vi "read TDMS file -- wavefront -- V1.vi"(6 "Data type":waveform(dbl), 7 "tdms file in":refnum<k34>, 9 "Data File Type":T2(ring), 10 "Data window":T1={"Start"=0, "Length"=500000, "Channel numbers"=[0], "Channel name"="Vpick", "Group name"="p"}, 11 "Input file path":path) -> (1 "1st channel length":u64=433333, 2 "Data out":waveform(dbl), 3 "Actual input file path":path, 5 "tdms file out":refnum<k34>)   [LabVIEW 2021]
uses:
  tdo -- new/Data window.ctl
panel:
  # "OR"
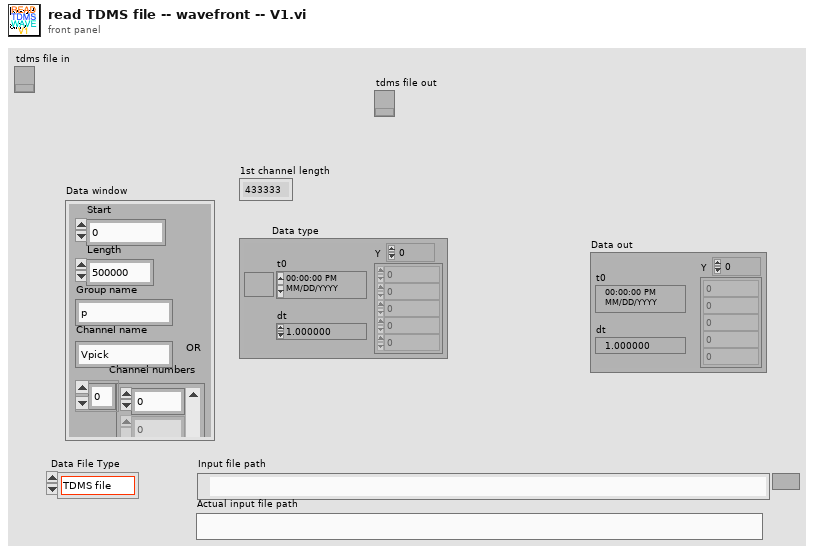
[diagram p1: front panel]
types:
  T1 = typedef "Data window.ctl" = cluster{"Start":i64, "Length":i64, "Channel numbers":i64[], "Channel name":string, "Group name":string}
  T2 = enum16{"TDMS file", "Tektronics ISF", "BinF file", "ASCII File", "BinH File", "BinW File", "BINARY File"}
  T3 = enum16{"open", "open or create", "create or replace", "create", "open (read-only)"}
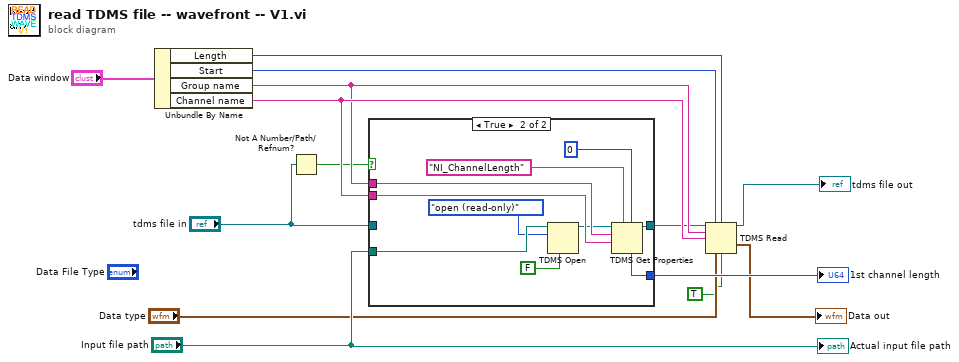
[diagram p0: block diagram]
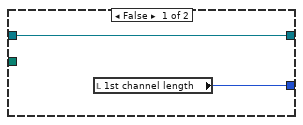
[diagram p2: hidden frame]
diagram:
  n1 = Unbundle By Name("Data window") -> ("Length"=w13:i64, "Start"=w4:i64, "Group name"=w10:string, "Channel name"=w12:string)
  n2 = Not A Number/Path/Refnum?(number/path/refnum="tdms file in") -> (NaN/Path/Refnum?=w2:bool)
  n3 = case shown="True" w2 {
    tunnel: [w16 w18] -> w3
    tunnel: "Input file path" -> [_ w26]
    tunnel: "tdms file in" -> [w16 _]
    tunnel: [w15 w22] -> w11
    tunnel: w12 -> [_ w21]
    tunnel: w10 -> [_ w20]
    frame False {
      n4 = local read "1st channel length"() -> (w15:u64)
    }
    frame True {
      n5 = TDMS Open(6:FALSE ("disable buffering (T)"), 10:T3."open (read-only)" ("operation (0:open)"), 11:w26) -> (3:w19:refnum<k34>)  [unwired: 4 in, 1 out]
      n6 = TDMS Get Properties(5:u64 0, 7:"NI_ChannelLength" ("property name"), 9:w21, 10:w20, 11:w19) -> (3:w18:refnum<k34>, 4:w22:u64)  [unwired: 1 in, 4 out]
    }
  }
  "1st channel length" <- w11
  n7 = TDMS Read(0:w3, 1:w4, 2:w13, 5:w10, 7:w12, 12:"Data type", 13:TRUE ("return channels in file order? (F)")) -> (4:→"tdms file out":refnum<k34>, 10:→"Data out":waveform(dbl))  [unwired: 1 in, 4 out]
  "Actual input file path" <- "Input file path"
